vi "poly1.vi"(6 "Minimum (-Inf,-Inf,-Inf)":cluster{"X":dbl, "Y":dbl, "Z":dbl}={"X"=-inf, "Y"=-inf, "Z"=-inf}, 7 "Maximum (Inf,Inf,Inf)":cluster{"X":dbl, "Y":dbl, "Z":dbl}={"X"=inf, "Y"=inf, "Z"=inf}, 8 "mask":cluster{"X":bool, "Y":bool, "Z":bool}, 9 "Translation (0,0,0)":cluster{"X":dbl, "Y":dbl, "Z":dbl}, 10 "Multiplier (1,1,1)":cluster{"X":dbl, "Y":dbl, "Z":dbl}={"X"=1.0, "Y"=1.0, "Z"=1.0}, 11 "input vector":cluster{"X":dbl, "Y":dbl, "Z":dbl}) -> (2 "In Range?":cluster{"X":bool, "Y":bool, "Z":bool}, 3 "output":cluster{"X":dbl, "Y":dbl, "Z":dbl})   [LabVIEW 2015]
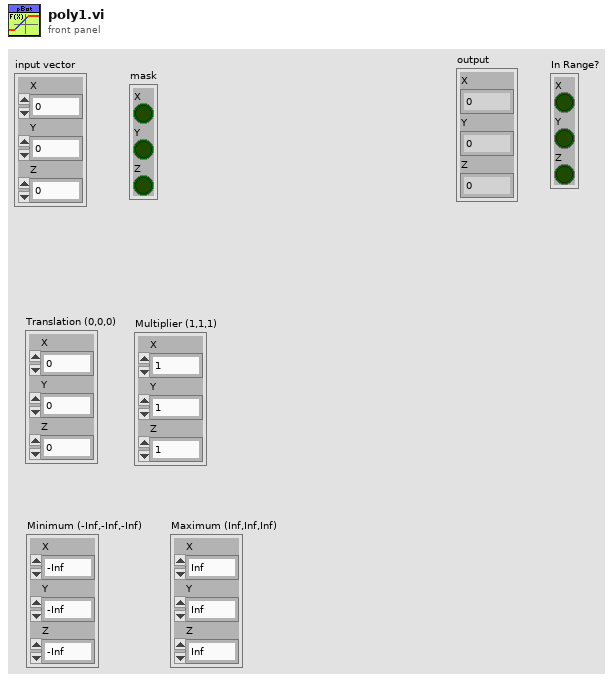
[diagram p1: front panel]
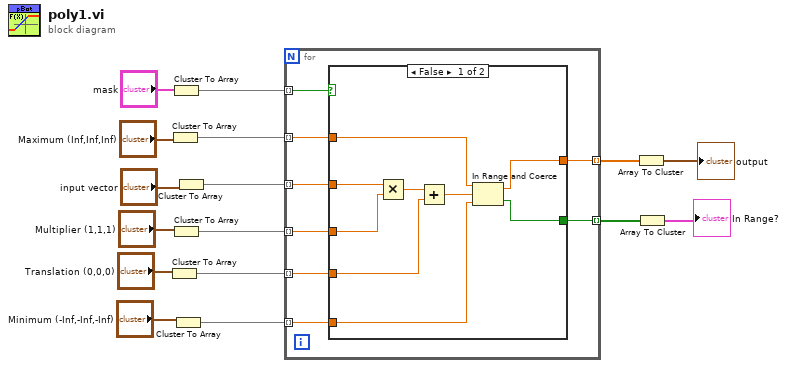
[diagram p0: block diagram]
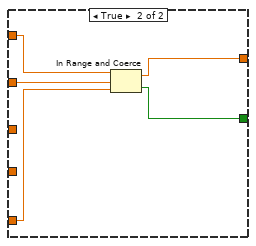
[diagram p2: hidden frame]
diagram:
  n1 = Cluster To Array(cluster="Translation (0,0,0)") -> (array=w8:dbl[])
  n2 = Cluster To Array(cluster="Maximum (Inf,Inf,Inf)") -> (array=w6:dbl[])
  n3 = Cluster To Array(cluster="mask") -> (array=w1:bool[])
  n4 = Cluster To Array(cluster="Multiplier (1,1,1)") -> (array=w9:dbl[])
  n5 = Cluster To Array(cluster="Minimum (-Inf,-Inf,-Inf)") -> (array=w7:dbl[])
  n6 = Cluster To Array(cluster="input vector") -> (array=w10:dbl[])
  n7 = for {
    tunnel: w10 -> [w24] mode=indexing
    tunnel: w9 -> [w23] mode=indexing
    tunnel: w8 -> [w22] mode=indexing
    tunnel: w7 -> [w21] mode=indexing
    tunnel: w6 -> [w20] mode=indexing
    tunnel: [w19] -> w5 mode=indexing
    tunnel: [w18] -> w3 mode=indexing
    tunnel: w1 -> [w17] mode=indexing
    n8 = case shown="False" w17 {
      tunnel: w24 -> [w31 w38]
      tunnel: w23 -> [w30 _]
      tunnel: w22 -> [w29 _]
      tunnel: w21 -> [w28 w36]
      tunnel: w20 -> [w27 w37]
      tunnel: [w26 w35] -> w19
      tunnel: [w25 w34] -> w18
      frame False {
        n9 = Multiply(x=w31, y=w30) -> (x*y=w33:dbl)
        n10 = Add(x=w33, y=w29) -> (x+y=w32:dbl)
        n11 = In Range and Coerce(upper limit=w27, x=w32, lower limit=w28) -> (coerced(x)=w26:dbl, In Range?=w25:bool)
      }
      frame True {
        n12 = In Range and Coerce(upper limit=w37, x=w38, lower limit=w36) -> (coerced(x)=w35:dbl, In Range?=w34:bool)
      }
    }
  }
  n13 = Array To Cluster(array=w5) -> (cluster=→"output":cluster{"[0]":dbl, "[1]":dbl, "[2]":dbl})
  n14 = Array To Cluster(array=w3) -> (cluster=→"In Range?":cluster{"[0]":bool, "[1]":bool, "[2]":bool})
